vi "DP-Plot DPGram Comparisons.vi"(0 "Plots":cluster{"I-O Plot":dbl[], "I-O Plot":dbl[]}[](array[cluster]), 1 "Plot refnum":refnum<vi>, 5 "Names":string[](array[string]), 11 "error in":errorcluster) -> (15 "error out":errorcluster)   [LabVIEW 2020]
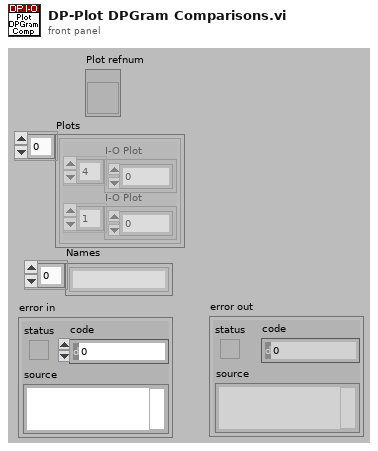
[diagram p1: front panel]
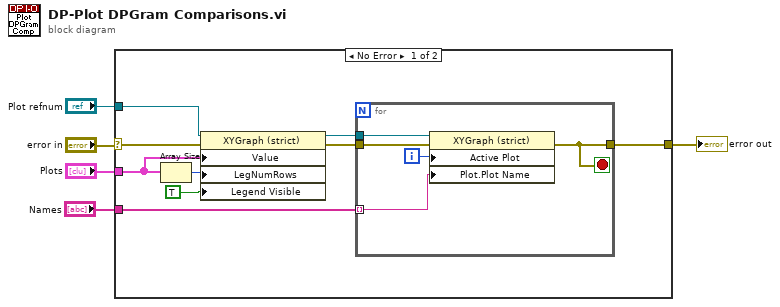
[diagram p0: block diagram]
diagram:
  n1 = case shown="No Error" "error in" {
    selector: "error in" -> [w11 w20]
    tunnel: "Plot refnum" -> [w14 _]
    tunnel: [w9 w20] -> w3
    tunnel: "Plots" -> [w8 _]
    tunnel: "Names" -> [w6 _]
    frame No Error {
      n2 = Array Size(array=w8) -> (size(s)=w12:i32)
      n3 = property class="XYGraph (strict)"(reference=w14, error in=w11, "Value"=w8, "LegNumRows"=w12, "Legend Visible"=TRUE ("Legend:Visible")) -> (reference out=w13:refnum<vi>, error out=w10:errorcluster)
      n4 = for {
        tunnel: w13 -> [w19]
        tunnel: w10 -> [w17]
        tunnel: [w16] -> w9
        tunnel: w6 -> [w15] mode=indexing
        i -> [w18]
        stop <- w16 stop-if-true
        n5 = property class="XYGraph (strict)"(reference=w19, error in=w17, "Active Plot"=w18, "Plot.Plot Name"=w15) -> (error out=w16:errorcluster)  [unwired: 1 out]
      }
    }
    frame Error {
    }
  }
  "error out" <- w3
